vi "4_2.vi"() -> ()   [LabVIEW 2020]
panel:
  in  "stop":bool
  out "Time elapsed":string
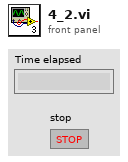
[diagram p1: front panel]
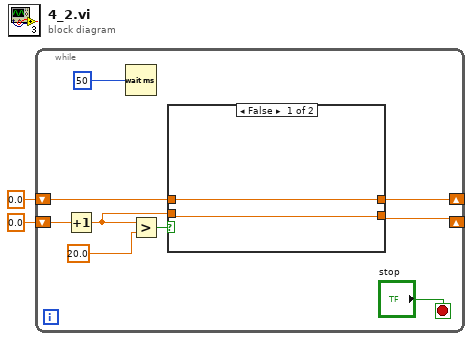
[diagram p0: block diagram]
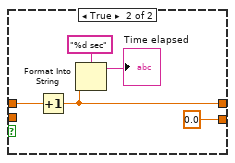
[diagram p2: hidden frame]
diagram:
  n1 = while {
    shift-right: [w6] -> _
    shift-left: 0.0 -> [w7]
    shift-right: [w4] -> _
    shift-left: 0.0 -> [w10]
    stop <- "stop" stop-if-true
    n2 = Increment(x=w10) -> (x+1=w5:dbl)
    n3 = Wait (ms)(milliseconds to wait=u32 50) -> ()  [unwired: 1 out]
    n4 = Greater?(x=w5, y=20.0) -> (0:w8:bool)
    n5 = case shown="False" w8 {
      tunnel: w7 -> [w13 w18]
      tunnel: [w13 w14] -> w6
      tunnel: w5 -> [w12 _]
      tunnel: [w12 0.0] -> w4
      frame False {
      }
      frame True {
        n6 = Increment(x=w18) -> (x+1=w14:dbl)
        n7 = Format Into String(format string="%d sec", w14) -> (resulting string=→"Time elapsed":string)  [unwired: 2 in, 1 out]
      }
    }
  }
